vi "Create All Message Queues.vi"(8 "error in (no error)":errorcluster) -> (0 "error out":errorcluster, 3 "Message Queues out":T1)   [LabVIEW 2014, in "Message Queue.lvlib"]
doc: "This VI creates and initializes all the message queues for your application. If your application requires more than one message queue, right-click the \"Message Queues\" constant above and select Open Type Def. Add the new Message Queue(s) to the type definition, then initialize them in this VI."
uses:
  Message Queue.lvlib
  All Message Queues.ctl
  Message Cluster.ctl
  Enqueue Message (Single).vi
panel:
  # "LICENSED MATERIALS – PROPERTY OF IBM\nCopyright IBM Corp. 2016,\nALL RIGHTS RESERVED"
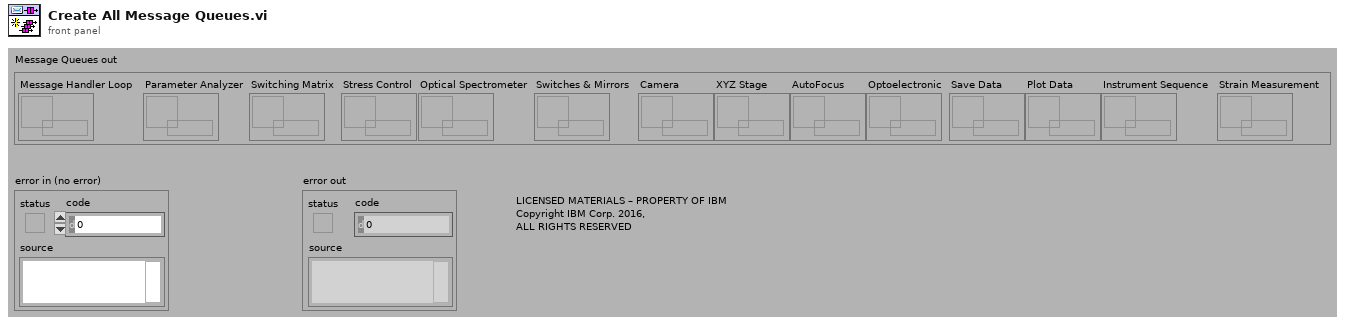
[diagram p1: front panel]
types:
  T1 = typedef "Message Queue.lvlib/All Message Queues.ctl" = cluster{"Message Handler Loop":refnum<queue>, "Parameter Analyzer":refnum<queue>, "Switching Matrix":refnum<queue>, "Stress Control":refnum<queue>, "Optical Spectrometer":refnum<queue>, "Switches & Mirrors":refnum<queue>, "Camera":refnum<queue>, "XYZ Stage":refnum<queue>, "AutoFocus":refnum<queue>, "Optoelectronic":refnum<queue>, "Save Data":refnum<queue>, "Plot Data":refnum<queue>, "Instrument Sequence":refnum<queue>, "Strain Measurement":refnum<queue>}
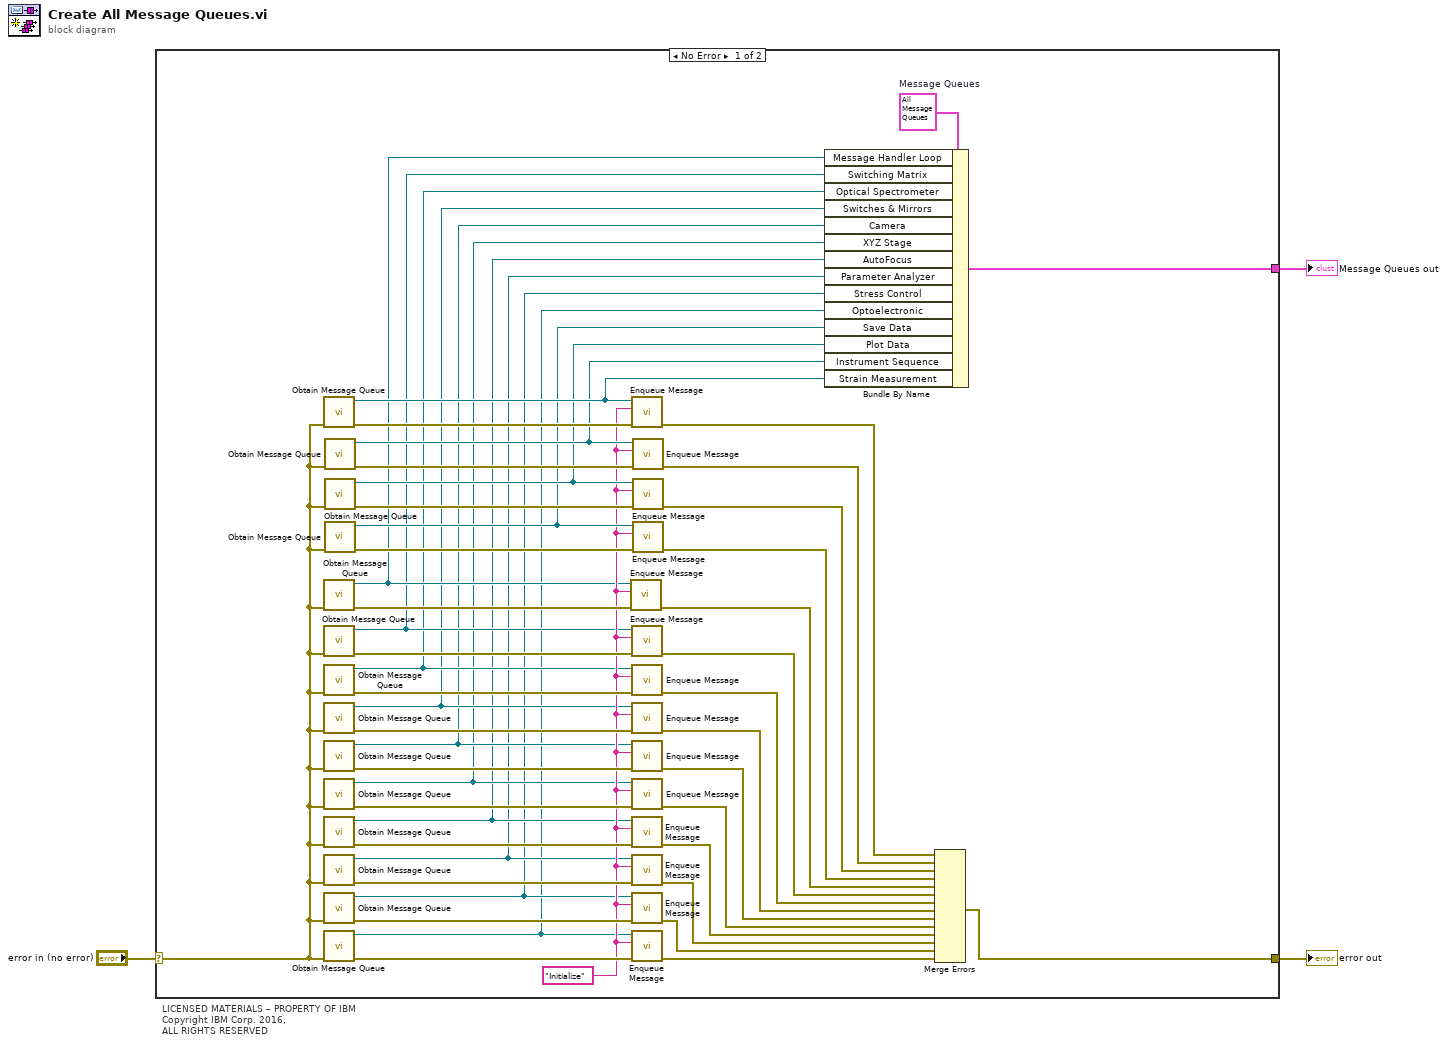
[diagram p0: block diagram]
diagram:
  # "LICENSED MATERIALS – PROPERTY OF IBM\nCopyright IBM Corp. 2016,\nALL RIGHTS RESERVED"
  n1 = case shown="No Error" "error in (no error)" {
    selector: "error in (no error)" -> [w14 w51]
    tunnel: [w20 w51] -> w3
    tunnel: [w48 _] -> w2
    frame No Error {
      w49 = T1 {"Message Handler Loop"=refnum, "Parameter Analyzer"=refnum, "Switching Matrix"=refnum, "Stress Control"=refnum, "Optical Spectrometer"=refnum, "Switches & Mirrors"=refnum, "Camera"=refnum, "XYZ Stage"=refnum, "AutoFocus"=refnum, "Optoelectronic"=refnum, "Save Data"=refnum, "Plot Data"=refnum, "Instrument Sequence"=refnum, "Strain Measurement"=refnum}  # Message Queues
      w15 = "Initialize" ("Message")
      n2 = call "Obtain Message Queue.vi"("error in (no error)"=w14) -> ("error out"=w25:errorcluster, "Message Queue"=w23:refnum<queue>)  [unwired: 1 in, 8 out]
      n3 = call "Obtain Message Queue.vi"("error in (no error)"=w14) -> ("error out"=w18:errorcluster, "Message Queue"=w13:refnum<queue>)  [unwired: 1 in, 8 out]
      n4 = call "Obtain Message Queue.vi"("error in (no error)"=w14) -> ("error out"=w32:errorcluster, "Message Queue"=w12:refnum<queue>)  [unwired: 1 in, 8 out]
      n5 = call "Obtain Message Queue.vi"("error in (no error)"=w14) -> ("error out"=w34:errorcluster, "Message Queue"=w11:refnum<queue>)  [unwired: 1 in, 8 out]
      n6 = call "Obtain Message Queue.vi"("error in (no error)"=w14) -> ("error out"=w47:errorcluster, "Message Queue"=w10:refnum<queue>)  [unwired: 1 in, 8 out]
      n7 = call "Obtain Message Queue.vi"("error in (no error)"=w14) -> ("error out"=w44:errorcluster, "Message Queue"=w9:refnum<queue>)  [unwired: 1 in, 8 out]
      n8 = call "Obtain Message Queue.vi"("error in (no error)"=w14) -> ("error out"=w43:errorcluster, "Message Queue"=w8:refnum<queue>)  [unwired: 1 in, 8 out]
      n9 = call "Obtain Message Queue.vi"("error in (no error)"=w14) -> ("error out"=w42:errorcluster, "Message Queue"=w7:refnum<queue>)  [unwired: 1 in, 8 out]
      n10 = call "Obtain Message Queue.vi"("error in (no error)"=w14) -> ("error out"=w41:errorcluster, "Message Queue"=w6:refnum<queue>)  [unwired: 1 in, 8 out]
      n11 = call "Obtain Message Queue.vi"("error in (no error)"=w14) -> ("error out"=w40:errorcluster, "Message Queue"=w5:refnum<queue>)  [unwired: 1 in, 8 out]
      n12 = call "Obtain Message Queue.vi"("error in (no error)"=w14) -> ("error out"=w46:errorcluster, "Message Queue"=w4:refnum<queue>)  [unwired: 1 in, 8 out]
      n13 = call "Obtain Message Queue.vi"("error in (no error)"=w14) -> ("error out"=w27:errorcluster, "Message Queue"=w22:refnum<queue>)  [unwired: 1 in, 8 out]
      n14 = call "Obtain Message Queue.vi"("error in (no error)"=w14) -> ("error out"=w29:errorcluster, "Message Queue"=w21:refnum<queue>)  [unwired: 1 in, 8 out]
      n15 = call "Obtain Message Queue.vi"("error in (no error)"=w14) -> ("error out"=w31:errorcluster, "Message Queue"=w19:refnum<queue>)  [unwired: 1 in, 8 out]
      n16 = call-poly "Enqueue Message.vi"("error in (no error)"=w18, "Message"=w15, "Message Queue"=w13) -> ("error out"=w16:errorcluster)  [unwired: 1 in, 7 out]
      n17 = call-poly "Enqueue Message.vi"("error in (no error)"=w25, "Message"=w15, "Message Queue"=w23) -> ("error out"=w24:errorcluster)  [unwired: 1 in, 7 out]
      n18 = call-poly "Enqueue Message.vi"("error in (no error)"=w32, "Message"=w15, "Message Queue"=w12) -> ("error out"=w17:errorcluster)  [unwired: 1 in, 7 out]
      n19 = call-poly "Enqueue Message.vi"("error in (no error)"=w34, "Message"=w15, "Message Queue"=w11) -> ("error out"=w33:errorcluster)  [unwired: 1 in, 7 out]
      n20 = call-poly "Enqueue Message.vi"("error in (no error)"=w47, "Message"=w15, "Message Queue"=w10) -> ("error out"=w50:errorcluster)  [unwired: 1 in, 7 out]
      n21 = call-poly "Enqueue Message.vi"("error in (no error)"=w44, "Message"=w15, "Message Queue"=w9) -> ("error out"=w39:errorcluster)  [unwired: 1 in, 7 out]
      n22 = call-poly "Enqueue Message.vi"("error in (no error)"=w43, "Message"=w15, "Message Queue"=w8) -> ("error out"=w38:errorcluster)  [unwired: 1 in, 7 out]
      n23 = call-poly "Enqueue Message.vi"("error in (no error)"=w42, "Message"=w15, "Message Queue"=w7) -> ("error out"=w35:errorcluster)  [unwired: 1 in, 7 out]
      n24 = call-poly "Enqueue Message.vi"("error in (no error)"=w41, "Message"=w15, "Message Queue"=w6) -> ("error out"=w36:errorcluster)  [unwired: 1 in, 7 out]
      n25 = call-poly "Enqueue Message.vi"("error in (no error)"=w40, "Message"=w15, "Message Queue"=w5) -> ("error out"=w37:errorcluster)  [unwired: 1 in, 7 out]
      n26 = call-poly "Enqueue Message.vi"("error in (no error)"=w46, "Message"=w15, "Message Queue"=w4) -> ("error out"=w45:errorcluster)  [unwired: 1 in, 7 out]
      n27 = call-poly "Enqueue Message.vi"("error in (no error)"=w27, "Message"=w15, "Message Queue"=w22) -> ("error out"=w26:errorcluster)  [unwired: 1 in, 7 out]
      n28 = call-poly "Enqueue Message.vi"("error in (no error)"=w29, "Message"=w15, "Message Queue"=w21) -> ("error out"=w28:errorcluster)  [unwired: 1 in, 7 out]
      n29 = call-poly "Enqueue Message.vi"("error in (no error)"=w31, "Message"=w15, "Message Queue"=w19) -> ("error out"=w30:errorcluster)  [unwired: 1 in, 7 out]
      n30 = Bundle By Name(cluster=w49, "Message Handler Loop"=w13, "Switching Matrix"=w12, "Optical Spectrometer"=w11, "Switches & Mirrors"=w10, "Camera"=w9, "XYZ Stage"=w8, "AutoFocus"=w7, "Parameter Analyzer"=w6, "Stress Control"=w5, "Optoelectronic"=w4, "Save Data"=w19, "Plot Data"=w21, "Instrument Sequence"=w22, "Strain Measurement"=w23) -> (w48:T1)
      n31 = Merge Errors(w24, w26, w28, w30, w16, w17, w33, w50, w39, w38, w35, w36, w37, w45) -> (w20:errorcluster)
    }
    frame Error {
    }
  }
  "Message Queues out" <- w2
  "error out" <- w3
